vi "Lossy Subscriber Test.vi"() -> ()   [LabVIEW 2013]
uses:
  Actor/src/Message/Lossy/FTW-Message-Lossy.lvclass
  Actor/src/Publisher/FTW-Publisher.lvclass
  Actor/src/Subscriber/FTW-Subscriber.lvclass
panel:
  out "Messages Received":i32
  out "Waveform Chart":cluster{i32, i32}(graph)
  in  "Holdoff Time":u32=1000
  in  "Holdoff":bool
  out "Message Body":string
  out "Message Header":string
  out "Sender Identity":string
  in  "Publisher Timeout":i32=100
  in  "Process Stop Button":bool
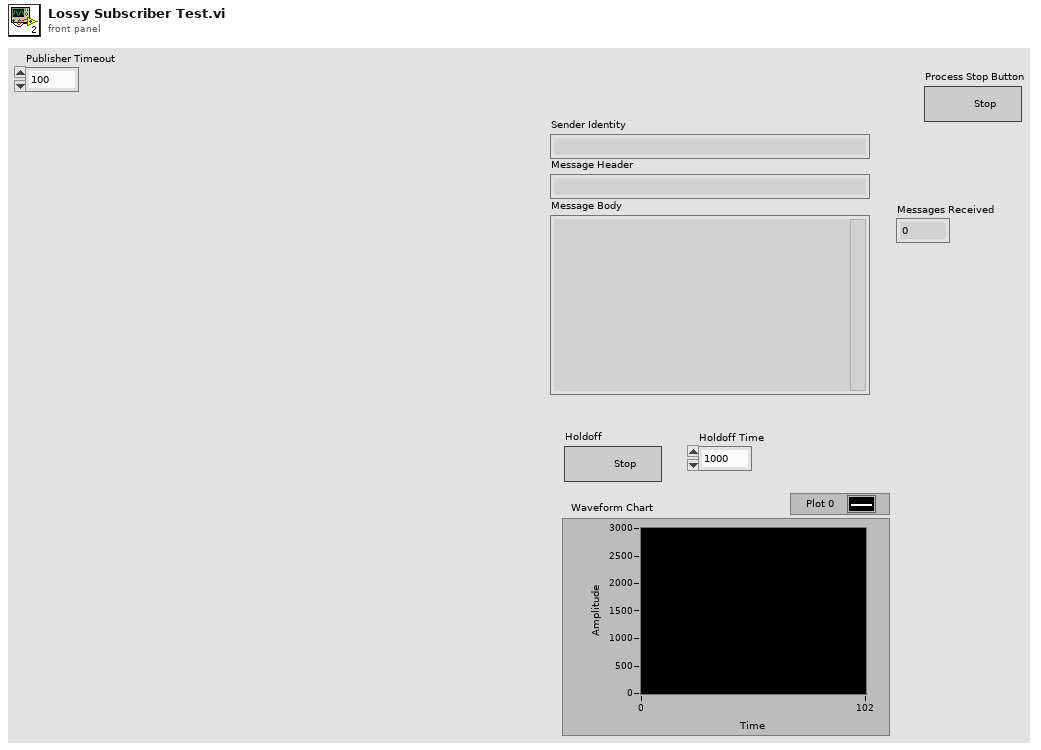
[diagram p1: front panel]
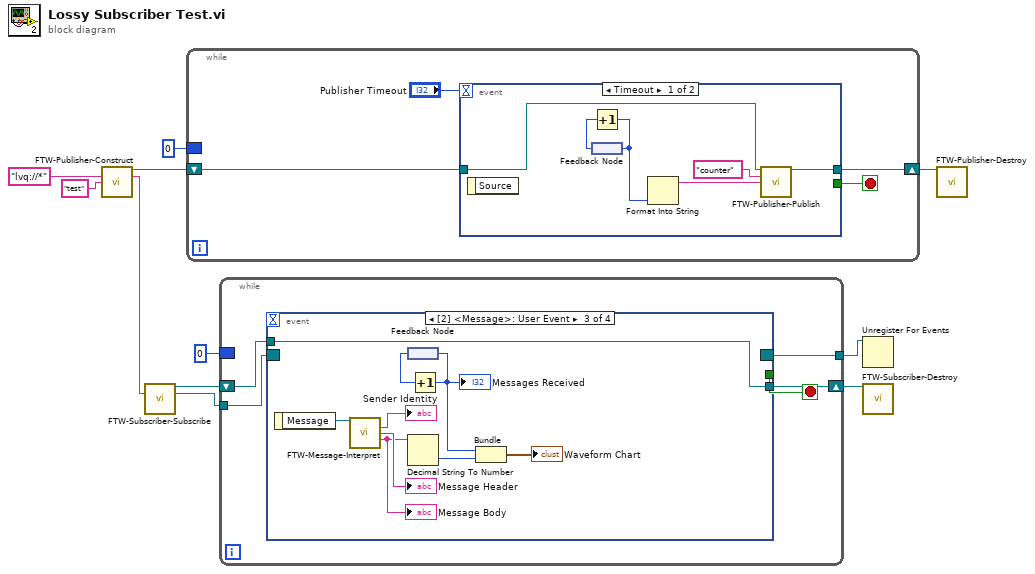
[diagram p0: block diagram]
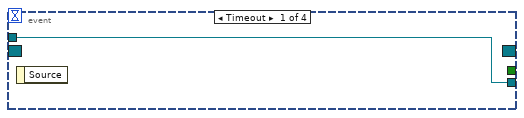
[diagram p2: hidden frame]
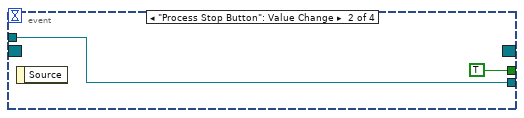
[diagram p3: hidden frame]
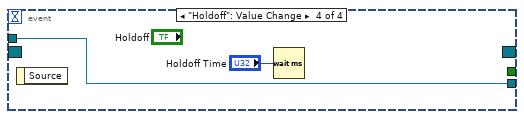
[diagram p4: hidden frame]
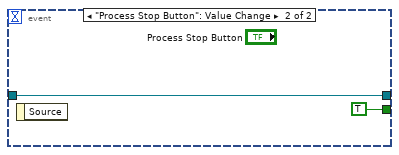
[diagram p5: hidden frame]
diagram:
  n1 = call "FTW-Publisher-Construct.vi"("Address"="lvq://*", "Identity"="test") -> ("FTW-Publisher Out"=w9:refnum<class "FTW-Publisher.lvclass">, "Actual Address"=w8:string)  [unwired: 11 in, 1 out]
  n2 = call "FTW-Subscriber-Subscribe.vi"("Addresses"=w8) -> ("FTW-Subscription Out"=w7:refnum<class "FTW-Subscriber.lvclass">, "Event Registration Refnum"=w4:refnum<event-registration>)  [unwired: 12 in, 1 out]
  n3 = while {
    shift-right: [w13] -> w5
    shift-left: w9 -> [w14]
    border: 0 -> [_]
    stop <- w15 stop-if-true
    n4 = event shown="[0] Timeout" {
      selector: _ -> [_ _]
      dyn-events: _ -> [_ _]
      timeout: "Publisher Timeout" -> [_ _]
      tunnel: [_ TRUE] -> w15
      tunnel: w14 -> [w21 w22]
      tunnel: [w20 w22] -> w13
      event Timeout {
        n5 = event-data() -> ()  [unwired: 1 in, 1 out]
        n6 = feedback #1() -> (w19:i32)
        n7 = Increment(x=w19) -> (x+1=w18:i32)
        n8 = feedback-in #1(w18) -> ()
        n9 = Format Into String(w18) -> (resulting string=w17:string)  [unwired: 3 in, 1 out]
        n10 = call "FTW-Publisher-Publish.vi"("FTW-Publisher In"=w21, "Header"="counter", "Body"=w17) -> ("FTW-Publisher Out"=w20:refnum<class "FTW-Publisher.lvclass">)  [unwired: 11 in, 1 out]
      }
      event "Process Stop Button": Value Change {
        n11 = event-data() -> ()  [unwired: 1 in, 1 out]
      }
    }
  }
  n12 = while {
    shift-right: [w26] -> w6
    shift-left: w7 -> [w27]
    tunnel: w4 -> [w25]
    tunnel: [w24] -> w3
    border: 0 -> [_]
    stop <- w28 stop-if-true
    n13 = event shown="[2] <Message>: User Event" {
      selector: w25 -> [_ _ _ _]
      dyn-events: [_ _ _ _] -> w24
      timeout: _ -> [_ _ _ _]
      tunnel: [_ TRUE _ _] -> w28
      tunnel: w27 -> [w29 w30 w40 w42]
      tunnel: [w29 w30 w40 w42] -> w26
      event Timeout {
        n14 = event-data() -> ()  [unwired: 1 in, 1 out]
      }
      event "Process Stop Button": Value Change {
        n15 = event-data() -> ()  [unwired: 1 in, 1 out]
      }
      event User Event {
        n16 = event-data() -> ("Message"=w39:refnum<class "FTW-Message-Lossy.lvclass">)  [unwired: 1 in]
        n17 = call-dynamic "FTW-Message-Interpret.vi"("FTW-Message-Lossy In"=w39) -> ("Sender Identity"=→"Sender Identity":string, "Message Header"=→"Message Header":string, "Message Body"=w36:string)  [unwired: 10 in, 2 out]
        "Message Body" <- w36
        n18 = feedback #2() -> (w34:i32)
        n19 = Decimal String To Number(string=w36) -> (number=w35:i32)  [unwired: 2 in, 1 out]
        n20 = Increment(x=w34) -> (x+1=w32:i32)
        "Messages Received" <- w32
        n21 = feedback-in #2(w32) -> ()
        n22 = Bundle(w32, w35) -> (→"Waveform Chart":cluster{i32, i32})  [unwired: 1 in]
      }
      event "Holdoff": Value Change {
        n23 = event-data() -> ()  [unwired: 1 in, 1 out]
        n24 = Wait (ms)(milliseconds to wait="Holdoff Time") -> ()  [unwired: 1 out]
      }
    }
  }
  n25 = Unregister For Events(event registration refnum=w3) -> ()  [unwired: 1 in, 1 out]
  n26 = call "FTW-Subscriber-Destroy.vi"("FTW-Subscription In"=w6) -> ()  [unwired: 14 in, 1 out]
  n27 = call "FTW-Publisher-Destroy.vi"("FTW-Publisher In"=w5) -> ()  [unwired: 14 in, 1 out]
